vi "Sending XY Data to Origin.vi"() -> ()   [LabVIEW 2020]
uses:
  Instance           5 33Saved   Sending XY Data to Origin .vi
  Instance           6 33Saved   Sending XY Data to Origin .vi
  Instance           7 33Saved   Sending XY Data to Origin .vi
panel:
  out "error out":errorcluster
  in  "X Value":i32
  in  "stop":bool
  out "XY Graph":cluster{"Y":dbl[], "Y":dbl[]}[](graph)
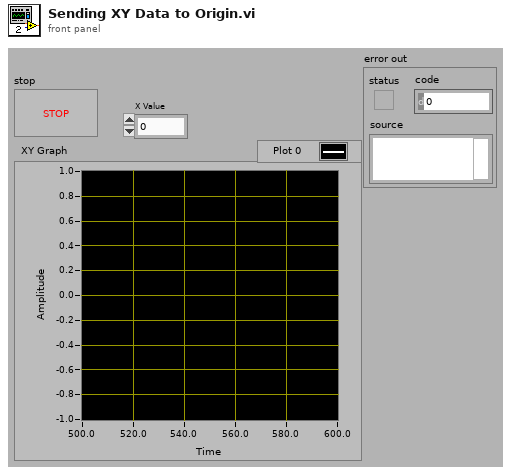
[diagram p1: front panel]
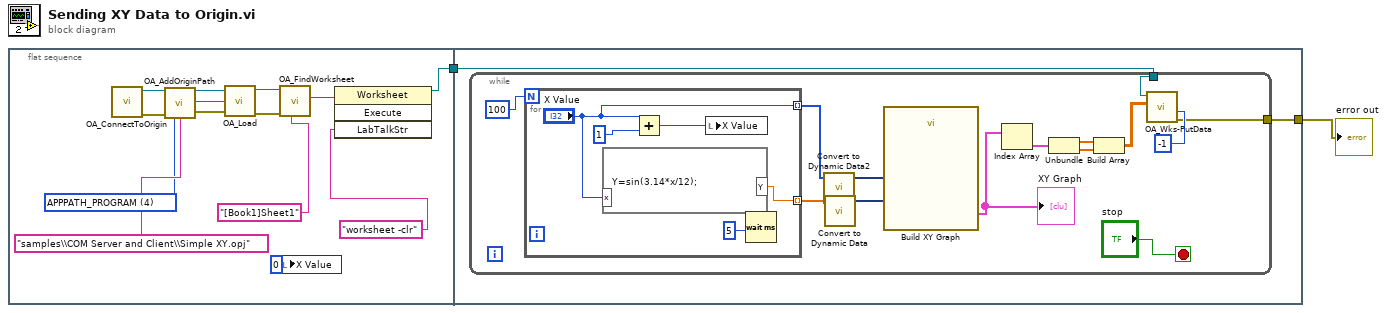
[diagram p0: block diagram]
diagram:
  n1 = flat-sequence {
    tunnel: [w4] -> w2
    tunnel: w2 -> [w18]
    tunnel: [w17] -> w1
    frame #0 {
      w8 = 4 items=["APPPATH_USER"=2, "APPPATH_GROUP"=3, "APPPATH_PROGRAM"=4] ("Type")
      n2 = call "OA_ConnectToOrigin.vi"() -> ("error out"=w11:errorcluster, "Origin.IOApplication"=w10:refnum<k7>)  [unwired: 8 in]
      n3 = call "OA_AddOriginPath.vi"("Origin.IOApplication"=w10, "error in (no error)"=w11, "Type"=w8, "Filename"="samples\\COM Server and Client\\Simple XY.opj" ("related path")) -> ("Origin.IOApplication"=w5:refnum<k7>, "path out"=w7:path, "error out"=w6:errorcluster)  [unwired: 9 in]
      n4 = call "OA_Load.vi"("error in (no error)"=w6, "Path"=w7, "Origin.IOApplication"=w5) -> ("error out"=w14:errorcluster, "Origin.IOApplication"=w13:refnum<k7>)  [unwired: 1 out]
      n5 = call "OA_FindWorksheet.vi"("Name"="[Book1]Sheet1", "error in (no error)"=w14, "Origin.IOApplication"=w13) -> ("Origin.Worksheet"=w15:refnum<k7>)  [unwired: 6 in, 2 out]
      n6 = local write "X Value"(0 ("X Value")) -> ()
      n7 = invoke class="Worksheet" method="Execute"(reference=w15, "LabTalkStr"="worksheet -clr") -> (reference out=w4:refnum<k7>)  [unwired: 2 in, 3 out]
    }
    frame #1 {
      n8 = while {
        tunnel: w18 -> [w20]
        tunnel: [w19] -> w17
        stop <- "stop" stop-if-true
        n9 = for {
          N: 100 -> [_]
          tunnel: [w37] -> w26 mode=indexing
          tunnel: ["X Value"] -> w21 mode=indexing
          n10 = formula code="Y=sin(3.14*x/12);"("x"="X Value") -> ("Y"=w37:dbl)
          n11 = Add(x="X Value", y=1) -> (x+y=w34:i32)
          n12 = local write "X Value"(w34) -> ()
          n13 = Wait (ms)(milliseconds to wait=u32 5) -> ()  [unwired: 1 out]
        }
        n14 = call "Convert to Dynamic Data2"("Array"=w21) -> ("Dynamic Data Type"=w23:dynamicdata)  [unwired: 3 in]
        n15 = call "Convert to Dynamic Data"("Array"=w26) -> ("Dynamic Data Type"=w25:dynamicdata)  [unwired: 3 in]
        n16 = call "Build XY Graph"("Y Input"=w25, "X Input"=w23) -> ("XY Graph"=w31:cluster{"Y":dbl[], "Y":dbl[]}[])  [unwired: 8 in, 1 out]
        "XY Graph" <- w31
        n17 = Index Array(array=w31) -> (element=w30:cluster{"Y":dbl[], "Y":dbl[]})  [unwired: 1 in]
        n18 = Unbundle(w30) -> ("Y"=w28:dbl[], "Y"=w29:dbl[])
        n19 = Build Array(w28, w29) -> (w27:dbl[][])
        n20 = call "OA_Wks-PutData.vi"("Row 1"=-1, "2d Data"=w27, "Origin.Worksheet"=w20) -> ("error out"=w19:errorcluster)  [unwired: 2 in, 2 out]
      }
    }
  }
  "error out" <- w1
